vi "Extract Chuck References.vi"(8 "error in":errorcluster, 10 "Slot":i32, 11 "Chuck Reference":refnum<vi>) -> (0 "error out":errorcluster, 2 "Serial Number Reference":refnum<vi>, 3 "Populated Button Reference":refnum<vi>)   [LabVIEW 2011]
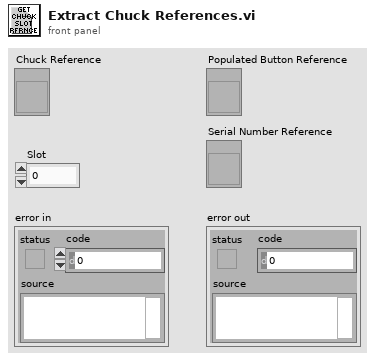
[diagram p1: front panel]
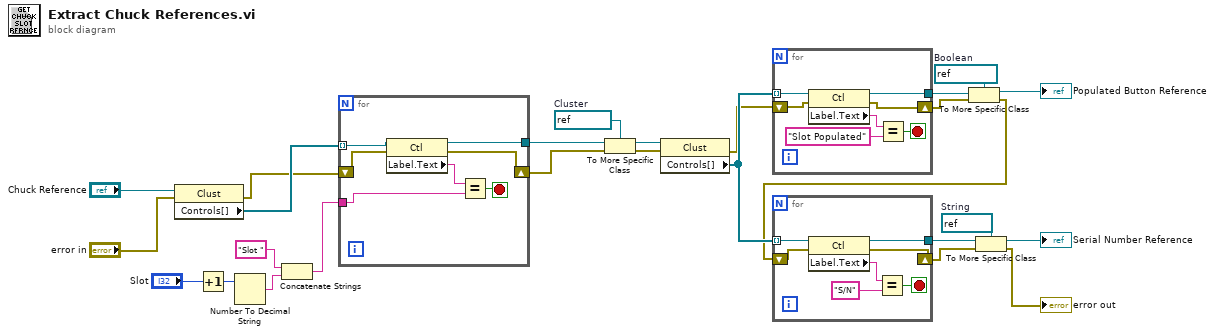
[diagram p0: block diagram]
diagram:
  w10 = refnum<vi> refnum  # String
  w12 = refnum<vi> refnum  # Boolean
  w20 = refnum<vi> refnum  # Cluster
  n1 = property class="Clust"(reference="Chuck Reference", error in="error in") -> (error out=w18:errorcluster, "Controls[]"=w24:refnum<vi>[])  [unwired: 1 out]
  n2 = Increment(x="Slot") -> (x+1=w2:i32)
  n3 = Number To Decimal String(number=w2) -> (decimal integer string=w23:string)  [unwired: 1 in]
  n4 = Concatenate Strings("Slot " ("y"), w23) -> (w21:string)
  n5 = for {
    tunnel: w24 -> [w33] mode=indexing
    tunnel: [w32] -> w19
    tunnel: w21 -> [w30]
    shift-right: [w27] -> w17
    shift-left: w18 -> [w28]
    stop <- w29 stop-if-true
    n6 = property class="Ctl"(reference=w33, error in=w28) -> (reference out=w32:refnum<vi>, error out=w27:errorcluster, "Label.Text"=w31:string)
    n7 = Equal?(x=w31, y=w30) -> (x = y?=w29:bool)
  }
  n8 = To More Specific Class(target class=w20, reference=w19, error in=w17) -> (specific class reference=w16:refnum<vi>, error out=w15:errorcluster)
  n9 = property class="Clust"(reference=w16, error in=w15) -> (error out=w7:errorcluster, "Controls[]"=w14:refnum<vi>[])  [unwired: 1 out]
  n10 = for {
    tunnel: w14 -> [w40] mode=indexing
    tunnel: [w39] -> w13
    shift-right: [w34] -> w6
    shift-left: w7 -> [w35]
    stop <- w36 stop-if-true
    n11 = property class="Ctl"(reference=w40, error in=w35) -> (reference out=w39:refnum<vi>, error out=w34:errorcluster, "Label.Text"=w38:string)
    n12 = Equal?(x=w38, y="Slot Populated") -> (x = y?=w36:bool)
  }
  n13 = To More Specific Class(target class=w12, reference=w13, error in=w6) -> (specific class reference=→"Populated Button Reference":refnum<vi>, error out=w5:errorcluster)
  n14 = for {
    tunnel: w14 -> [w47] mode=indexing
    tunnel: [w46] -> w9
    shift-right: [w41] -> w4
    shift-left: w5 -> [w42]
    stop <- w44 stop-if-true
    n15 = property class="Ctl"(reference=w47, error in=w42) -> (reference out=w46:refnum<vi>, error out=w41:errorcluster, "Label.Text"=w43:string)
    n16 = Equal?(x=w43, y="S/N") -> (x = y?=w44:bool)
  }
  n17 = To More Specific Class(target class=w10, reference=w9, error in=w4) -> (specific class reference=→"Serial Number Reference":refnum<vi>, error out=→"error out":errorcluster)
